vi "CheckShot2Boundary.vi"(6 "IntensityArray_IN":u8[][](array[numeric]), 11 "ShotArray_IN":T1[](array[typedef])) -> (3 "ShotArray_OUT":T1[](array[typedef]), 4 "IntensityArray_OUT":u8[][](array[numeric]))   [LabVIEW 2022 SP3]
uses:
  ShotCluster.ctl
  move_dir_ud.ctl
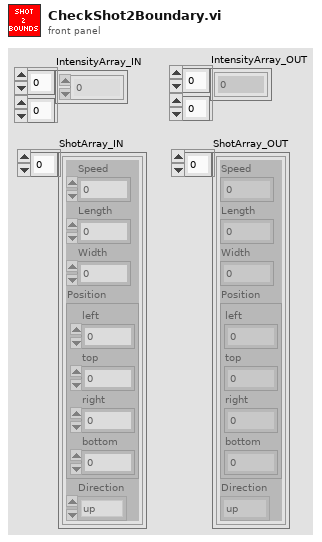
[diagram p1: front panel]
types:
  T1 = typedef "ShotCluster.ctl" = cluster{"Speed":u32, "Length":u32, "Width":u32, "Position":cluster{"left":i16, "top":i16, "right":i16, "bottom":i16}, "Direction":T2}
  T2 = typedef "move_dir_ud.ctl" = enum16{"up", "down"}
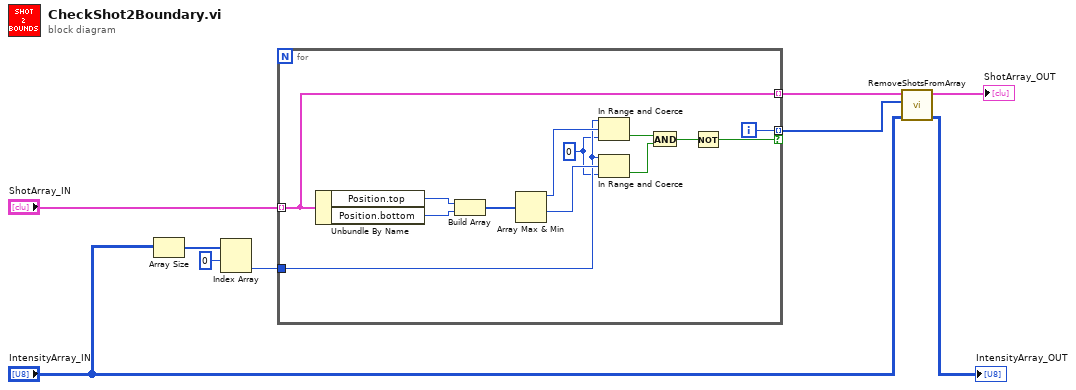
[diagram p0: block diagram]
diagram:
  n1 = Array Size(array="IntensityArray_IN") -> (size(s)=w8:i32[])
  n2 = Index Array(array=w8, index #1=0 ("index")) -> (element #2=w6:i32)  [unwired: 1 in, 1 out]
  n3 = for {
    tunnel: "ShotArray_IN" -> [w13] mode=indexing
    tunnel: w6 -> [w17]
    tunnel: [w13] -> w5 mode=indexing
    tunnel: [w12] -> w1 mode=indexing if=w10
    i -> [w12]
    w16 = 0 ("lower limit")
    n4 = Unbundle By Name(w13) -> ("Position.top"=w22:i16, "Position.bottom"=w21:i16)
    n5 = Build Array(w22, w21) -> (w20:i16[])
    n6 = Array Max & Min(array=w20) -> (max value=w19:i16, min value=w18:i16)  [unwired: 2 out]
    n7 = In Range and Coerce(upper limit=w17, x=w19, lower limit=w16) -> (In Range?=w15:bool)  [unwired: 1 out]
    n8 = In Range and Coerce(upper limit=w17, x=w18, lower limit=w16) -> (In Range?=w14:bool)  [unwired: 1 out]
    n9 = And(x=w15, y=w14) -> (x .and. y?=w11:bool)
    n10 = Not(x=w11) -> (.not. x?=w10:bool)
  }
  n11 = call "RemoveShotsFromArray.vi"("IntensityArray_IN"="IntensityArray_IN", "Indexes"=w1, "ShotArray_IN"=w5) -> ("IntensityArray_OUT"=→"IntensityArray_OUT":u8[][], "ShotArray_OUT"=→"ShotArray_OUT":T1[])  [unwired: 7 in]
